vi "remove_edge.vi"(10 "edge":refnum<class "Edge.lvclass">, 11 "digraph":refnum<class "DiGraph.lvclass">) -> (2 "edge not found?":bool, 3 "digraph out":refnum<class "DiGraph.lvclass">)   [LabVIEW 2020, in "graph.lvlib" / "DiGraph.lvclass"]
uses:
  DiGraph.lvclass
  Edge/Edge.lvclass
  DiGraph.lvclass/DiGraph.ctl
  Graph/Graph.lvclass
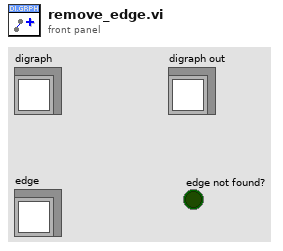
[diagram p1: front panel]
types:
  T1 = typedef "edge-definition-cluster.ctl" = cluster{"source-id":refnum<class "ID.lvclass">, "sink-id":refnum<class "ID.lvclass">}
  T2 = map{refnum<class "ID.lvclass">, set{refnum<class "ID.lvclass">}}
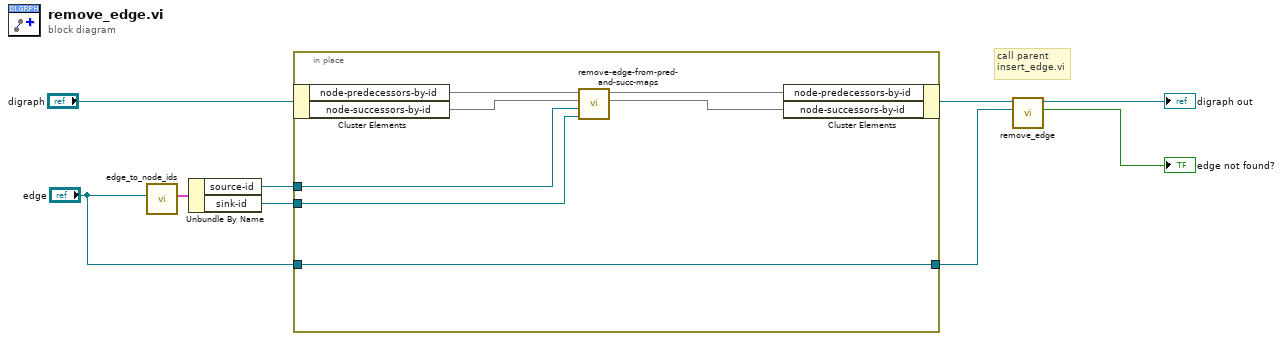
[diagram p0: block diagram]
diagram:
  # "call parent\ninsert_edge.vi"
  n1 = call "edge_to_node_ids.vi"("edge"="edge") -> ("node-ids-cluster"=w4:T1)  [unwired: 10 in]
  n2 = Unbundle By Name(w4) -> ("source-id"=w3:refnum<class "ID.lvclass">, "sink-id"=w1:refnum<class "ID.lvclass">)
  n3 = in-place {
    in-place-border: "edge" -> [w15]
    in-place-border: [w15] -> w6
    in-place-border: w3 -> [w13]
    in-place-border: w1 -> [w10]
    n4 = in-place-cluster #1("digraph") -> ("node-predecessors-by-id"=w14:T2, "node-successors-by-id"=w12:T2)
    n5 = call "remove-edge-from-pred-and-succ-maps.vi"("sink-id"=w10, "source-id"=w13, "node-successors-by-id"=w12, "node-predecessors-by-id"=w14) -> ("node-successors-by-id out"=w11:T2, "node-predecessors-by-id out"=w16:T2)  [unwired: 6 in]
    n6 = in-place-cluster #1("node-predecessors-by-id"=w16, "node-successors-by-id"=w11) -> (w8:refnum<class "DiGraph.lvclass">)
  }
  n7 = call-parent "remove_edge.vi"("edge"=w6, "graph"=w8) -> ("key not found?"=→"edge not found?":bool, "graph out"=→"digraph out":refnum<class "DiGraph.lvclass">)  [unwired: 8 in]
